vi "AutoTurnGyro.vi"(7 "Sensor (Gyro)":enum16{"Gyro", "Vision"}(ring), 8 "error in":errorcluster, 10 "Turn Amount":i32=45, 11 "Initial Angle":dbl) -> (0 "error out":errorcluster, 3 "Target Angle Out":dbl)   [LabVIEW 2012]
doc: "This VI is called when autonomous begins, and will automatically be terminated when autonomous ends. You can carry out timed or sensor driven robot movement independently without needing to return to the caller."
uses:
  <vilib>/Rock Robotics/WPI/RobotDrive/WPI_RobotDriveGetSetRefNum.vi
  Robot Global Data.vi
  <vilib>/addons/control/pid/NI_PID_pid.lvlib
  <vilib>/addons/control/pid/pid.llb/PID (DBL).vi
  <vilib>/addons/control/pid/pid.llb/PID Structure Conversion (DBL).vi
panel:
  out "Loop (Hz)":dbl
  out "Output":dbl
  in  "PID gains":T1={"proportional gain (Kc)"=0.012000000000000004, "integral time (Ti, min)"=0.035, "derivative time (Td, min)"=0.0009} {"proportional gain (Kc)" format="%_6f"; "integral time (Ti, min)" format="%_6f"; "derivative time (Td, min)" format="%_6f"}
  out "Graph":cluster{dbl, dbl, "Time for happy (ms)":dbl}(graph)
  out "PID Output":dbl format="%.2f"
  out "Error":dbl
  out "Current Angle":dbl
  # "Low gear\nMax turn - 0.71\nMin turn - 0.45"
  # "Curve Value Input Not used when using Gyro"
  # "\"-\" Turns Left\n\"+\" Turns Right"
  # "If Using Gyro:\nEnter Turn amount in Degrees:\n\"-\" AngleTurns Left\n\"+\" Angle Turns Right"
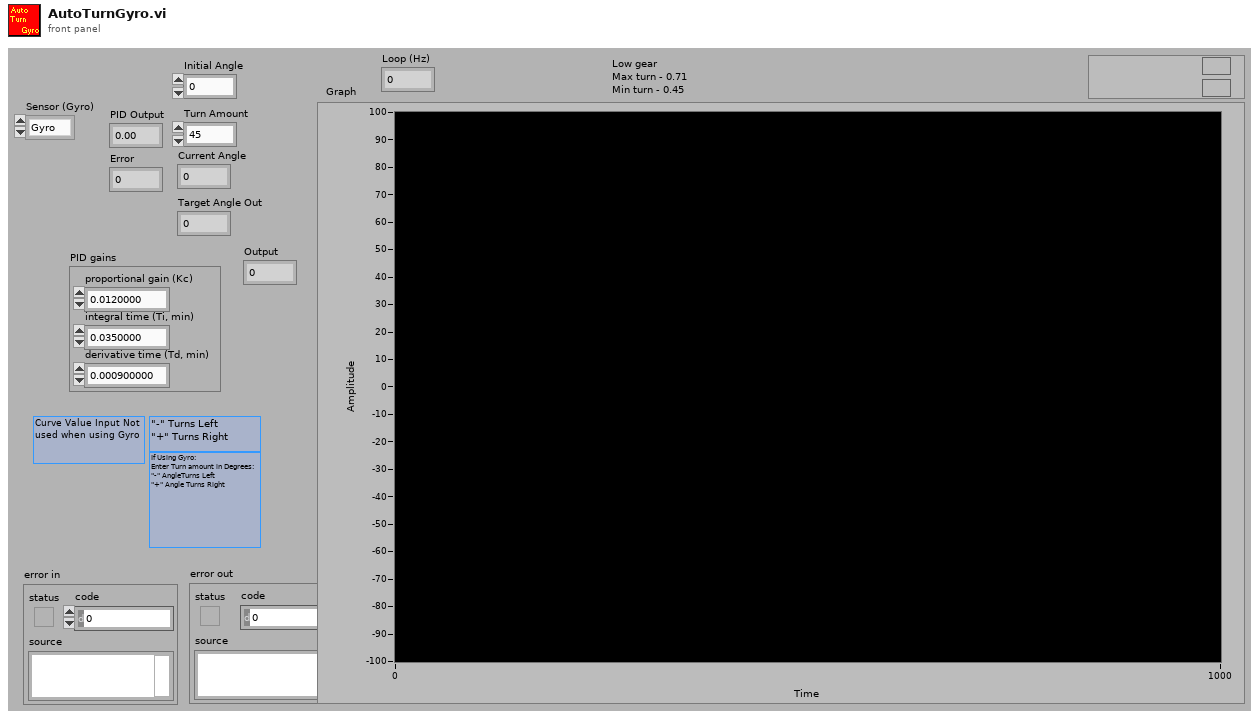
[diagram p1: front panel]
types:
  T1 = cluster{"proportional gain (Kc)":dbl, "integral time (Ti, min)":dbl, "derivative time (Td, min)":dbl}
  T2 = typedef "WPI_RobotDriveDevRef.ctl" = cluster{"DevStatus":errorcluster, "Motors[]":T3[], "Square Inputs":bool, "Max Output":dbl, "Isochronous":bool}
  T3 = typedef "WPI_MotorControlDeviceRef.ctl" = cluster{"DeviceStatus":errorcluster, "Type":enum16{"PWM", "CAN"}, "PWM":cluster{"Digital Module":T4, "PWM Channel":T5, "DeadBand":T6}, "CAN":cluster{"Device Number":u8, "Control Mode":T7, "Semaphore":T8, "Max Vout":dbl}, "Invert":bool, "TransformRef":T9, "InvTransformRef":T9}
  T4 = typedef "FPGA_TypedefDigitalModule.ctl" = enum16{"Digital Module 1", "Digital Module 2"}
  T5 = typedef "FPGA_DIOPWMChannel.ctl" = enum8{"PWM 1", "PWM 2", "PWM 3", "PWM 4", "PWM 5", "PWM 6", "PWM 7", "PWM 8", "PWM 9", "PWM 10", "Invalid"}
  T6 = typedef "WPI_PWMDeadband.ctl" = cluster{"Name":string, "maxPositivePwm":i32, "minPositivePwm":i32, "centerPwm":i32, "maxNegativePwm":i32, "minNegativePwm":i32, "angularRange":u16}
  T7 = typedef "WPI_CANJaguar_ControlMode.ctl" = enum8{"Percent VBus", "Current", "Speed", "Position", "Voltage"}
  T8 = typedef "Semaphore RefNum" = refnum<k1>
  T9 = typedef "WPI_PWMTransform_ConPane.ctl" = refnum<vi>
  T10 = typedef "WPI_GyroDevRef.ctl" = cluster{"DevStatus":errorcluster, "Analog Module":T11, "Analog Channel":T12, "Offset":dbl, "Gain (VoltsPerDegree/Second)":dbl}
  T11 = typedef "FPGA_TypedefAnalogModule.ctl" = enum16{"Analog Module 1", "Analog Module 2"}
  T12 = typedef "FPGA_AIChannel.ctl" = enum8{"AI 1", "AI 2", "AI 3", "AI 4", "AI 5", "AI 6", "AI 7", "AI 8", "Invalid"}
  T13 = enum16{"Academic (Standard)", "Parallel", "Series"}
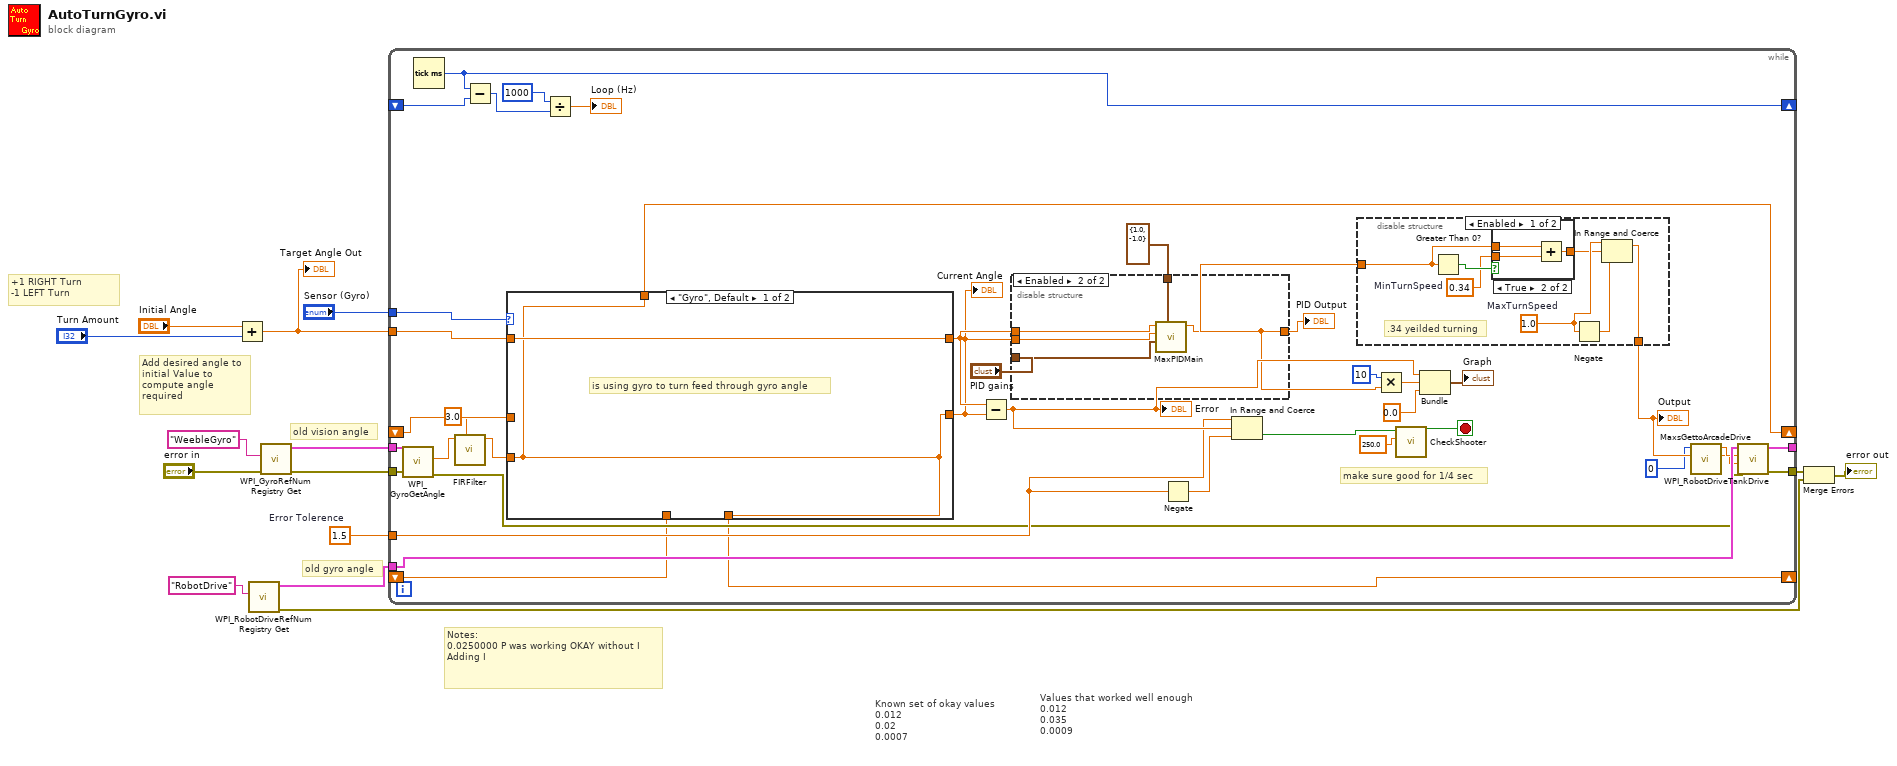
[diagram p0: block diagram]
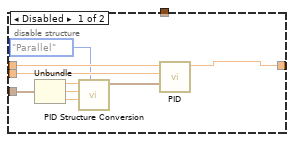
[diagram p2: hidden frame]
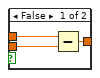
[diagram p3: hidden frame]
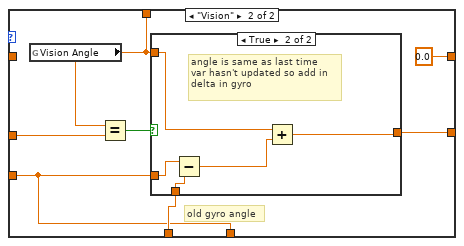
[diagram p5: hidden frame]
diagram:
  w9 = 1.5  # Error Tolerence
  # "Values that worked well enough\n0.012\n0.035\n0.0009"
  # "Known set of okay values\n0.012\n0.02\n0.0007"
  # "Notes:\n0.0250000 P was working OKAY without I\nAdding I"
  # "old vision angle"
  # "old gyro angle"
  # "+1 RIGHT Turn\n-1 LEFT Turn"
  # "Add desired angle to initial Value to\ncompute angle required"
  n1 = Add(x="Initial Angle", y="Turn Amount") -> (x+y=w3:dbl)
  "Target Angle Out" <- w3
  n2 = call <vilib>:"WPI_RobotDriveRefNum Registry Get.vi"("refnum name"="RobotDrive") -> ("error out"=w4:errorcluster, "RobotDriveDevRef"=w6:T2)  [unwired: 9 in]
  n3 = call <vilib>:"WPI_GyroRefNum Registry Get.vi"("error in (no error)"="error in", "refnum name"="WeebleGyro") -> ("error out"=w7:errorcluster, "GyroDevRef"=w8:T10)  [unwired: 8 in]
  n4 = while {
    tunnel: [w53] -> _
    tunnel: [w52] -> w5
    tunnel: "Sensor (Gyro)" -> [w50]
    tunnel: w9 -> [w47]
    tunnel: w8 -> [w39]
    tunnel: w7 -> [w38]
    tunnel: w6 -> [w46]
    tunnel: w3 -> [w45]
    shift-right: [w34] -> _
    shift-left: _ -> [w40]
    shift-right: [w36] -> _
    shift-left: _ -> [w35]
    shift-right: [w22] -> _
    shift-left: _ -> [w21]
    stop <- w33 stop-if-true
    # "make sure good for 1/4 sec"
    n5 = call <vilib>:"WPI_GyroGetAngle.vi"("error in (no error)"=w38, "GyroDevRef"=w39) -> ("error out"=w37:errorcluster, "Angle"=w16:dbl)  [unwired: 8 out]
    n6 = Tick Count (ms)() -> (millisecond timer value=w22:u32)
    n7 = call "FIRFilter.vi"("Filter Size"=3.0, "Input"=w16) -> ("Output"=w17:dbl)  [unwired: 9 in]
    n8 = Subtract(x=w22, y=w21) -> (x-y=w20:u32)
    n9 = case shown="\"Gyro\", Default" w50 {
      tunnel: [w83 w90] -> w41
      tunnel: w45 -> [w84 _]
      tunnel: [w84 0.0] -> w44
      tunnel: w40 -> [_ w85]
      tunnel: w17 -> [w83 w87]
      tunnel: [w83 w87] -> w36
      tunnel: w35 -> [_ w88]
      tunnel: [w83 w86] -> w34
      frame "Gyro", Default {
        # "is using gyro to turn feed through gyro angle"
      }
      frame "Vision" {
        # "old gyro angle"
        n10 = global read "Robot Global Data.vi" "Vision Angle"() -> (w86:dbl)
        n11 = Equal?(x=w86, y=w85) -> (x = y?=w89:bool)
        n12 = case shown="True" w89 {
          tunnel: [w92 w93] -> w90
          tunnel: w86 -> [w92 w95]
          tunnel: w88 -> [_ w96]
          tunnel: w87 -> [_ w97]
          frame False {
            # "if vision angle isn't the same\nas last time. this means it updated\nand is good to use"
          }
          frame True {
            # "angle is same as last time\nvar hasn't updated so add in\ndelta in gyro"
            n13 = Subtract(x=w97, y=w96) -> (x-y=w94:dbl)
            n14 = Add(x=w95, y=w94) -> (x+y=w93:dbl)
          }
        }
      }
    }
    "Current Angle" <- w41
    n15 = Divide(x=1000, y=w20) -> (x/y=→"Loop (Hz)":dbl)
    n16 = Subtract(x=w44, y=w41) -> (x-y=w49:dbl)
    "Error" <- w49
    n17 = disable-structure shown="Enabled" {
      disable-tunnel: w44 -> [w62 w67]
      disable-tunnel: w41 -> [w61 w66]
      disable-tunnel: [w60 w68] -> w27
      disable-tunnel: "PID gains" -> [w57 w64]
      disable-tunnel: cluster{"output high":dbl, "output low":dbl} {"output high"=1.0, "output low"=-1.0} ("output range") -> [_ w65]
      frame Disabled {
        n18 = Unbundle(w57) -> ("proportional gain (Kc)"=w56:dbl, "integral time (Ti, min)"=w55:dbl, "derivative time (Td, min)"=w54:dbl)
        n19 = call-poly <vilib>:"PID Structure Conversion.vi"("PID structure"=T13."Parallel", "derivative"=w54, "integral"=w55, "proportional"=w56) -> ("PID gains"=w59:T1)  [unwired: 7 in]
        n20 = call-poly <vilib>:"PID.vi"("PID gains"=w59, "process variable"=w61, "setpoint"=w62) -> ("output"=w60:dbl, "output range"=w63:cluster{"output high":dbl, "output low":dbl})  [unwired: 2 in, 5 out]
      }
      frame Enabled {
        n21 = call "MaxPIDMain.vi"("Output Range"=w65, "PID gains"=w64, "process variable"=w66, "setpoint"=w67) -> ("Output"=w68:dbl)  [unwired: 6 in, 1 out]
      }
    }
    "PID Output" <- w27
    n22 = Negate(x=w47) -> (-x=w48:dbl)
    n23 = In Range and Coerce(upper limit=w47, x=w49, lower limit=w48) -> (In Range?=w32:bool)  [unwired: 1 out]
    n24 = disable-structure shown="Enabled" {
      disable-tunnel: [w75 w82] -> w24
      disable-tunnel: w27 -> [w69 w82]
      frame Enabled {
        w73 = 1.0  # MaxTurnSpeed
        w70 = 0.34  # MinTurnSpeed
        # ".34 yeilded turning"
        n25 = Greater Than 0?(x=w69) -> (x > 0?=w71:bool)
        n26 = case shown="True" w71 {
          tunnel: [w77 w81] -> w72
          tunnel: w69 -> [w78 w80]
          tunnel: w70 -> [w76 w79]
          frame False {
            n27 = Subtract(x=w78, y=w76) -> (x-y=w77:dbl)
          }
          frame True {
            n28 = Add(x=w80, y=w79) -> (x+y=w81:dbl)
          }
        }
        n29 = Negate(x=w73) -> (-x=w74:dbl)
        n30 = In Range and Coerce(upper limit=w73, x=w72, lower limit=w74) -> (coerced(x)=w75:dbl)  [unwired: 1 out]
      }
      frame Disabled {
      }
    }
    "Output" <- w24
    n31 = Multiply(x=10, y=w27) -> (x*y=w43:dbl)
    n32 = call "CheckShooter.vi"("Time for happy (ms)"=250.0, "Shooter Good?"=w32) -> ("Good to shoot"=w33:bool)  [unwired: 9 in]
    n33 = Bundle(w49, w43, "Time for happy (ms)"=0.0) -> (→"Graph":cluster{dbl, dbl, "Time for happy (ms)":dbl})  [unwired: 1 out]
    n34 = call "MaxsGettoArcadeDrive.vi"("Driver X In"=w24, "Driver Y In"=0) -> ("Right Out"=w25:dbl, "Left Out"=w26:dbl)  [unwired: 8 in]
    n35 = call <vilib>:"WPI_RobotDriveTankDrive.vi"("error in (no error)"=w37, "Right axis value"=w25, "Left axis value"=w26, "RobotDriveDevRef"=w46) -> ("error out"=w52:errorcluster, "RobotDriveDevRef"=w53:T2)  [unwired: 5 in, 1 out]
  }
  n36 = Merge Errors(w5, w4) -> (→"error out":errorcluster)
